vi "File IO - Save Test Parameters to File.vi"(8 "error in":errorcluster, 10 "Experiment Parameter Values (default)":T1(array[cluster]), 11 "start path":path=path "") -> (0 "error out":errorcluster, 3 "selected path":path)   [LabVIEW 2014, in "Core SubVIs.lvlib"]
uses:
  Core SubVIs.lvlib
  Instance           1 46Saved   File IO - Save Test Parameters to File .vi
  <vilib>/Utility/config.llb/Write Key (String).vi
  <vilib>/Utility/config.llb/NI_LVConfig.lvlib
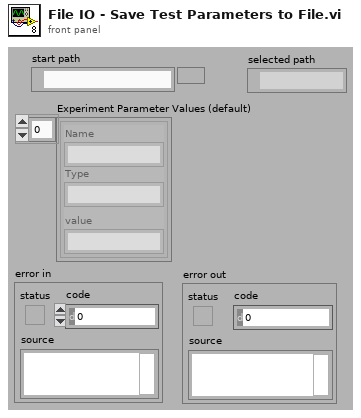
[diagram p1: front panel]
types:
  T1 = cluster{"Name":string, "Type":string, "value":string}[]
  T2 = typedef "NI_LVConfig.lvlib/Config Data RefNum.ctl" = refnum<k1>
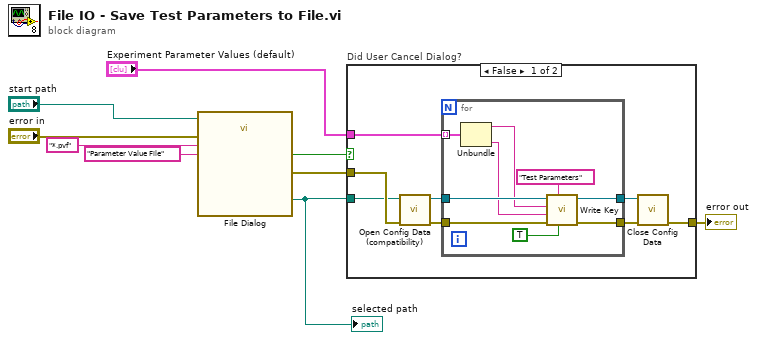
[diagram p0: block diagram]
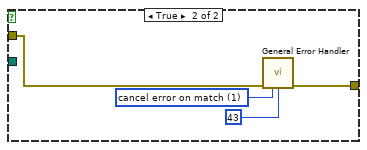
[diagram p2: hidden frame]
diagram:
  n1 = call "File Dialog"("start path"="start path", "error in"="error in", "pattern (all files)"="*.pvf", "pattern label"="Parameter Value File") -> ("selected path"=w6:path, "cancelled"=w5:bool, "error out"=w3:errorcluster)  [unwired: 3 in, 6 out]
  "selected path" <- w6
  n2 = case "Did User Cancel Dialog?" shown="False" w5 {
    tunnel: w6 -> [w15 _]
    tunnel: "Experiment Parameter Values (default)" -> [w17 _]
    tunnel: w3 -> [w16 w30]
    tunnel: [w10 w29] -> w2
    frame False {
      n3 = call <vilib>:"Open Config Data (compatibility).vi"("error in (no error)"=w16, "configuration file path"=w15) -> ("error out"=w13:errorcluster, "refnum"=w14:T2)  [unwired: 7 in, 1 out]
      n4 = for {
        tunnel: w17 -> [w26] mode=indexing
        tunnel: w14 -> [w25]
        tunnel: w13 -> [w24]
        tunnel: [w19] -> w11
        tunnel: [w18] -> w12
        n5 = Unbundle(w26) -> ("Name"=w22:string, "value"=w21:string)  [unwired: 1 out]
        n6 = call-poly <vilib>:"Write Key.vi"("write raw string? (F)"=TRUE, "section"="Test Parameters", "error in (no error)"=w24, "value"=w21, "key"=w22, "refnum"=w25) -> ("error out"=w18:errorcluster, "refnum out"=w19:T2)  [unwired: 4 out]
      }
      n7 = call <vilib>:"Close Config Data.vi"("error in (no error)"=w12, "refnum"=w11) -> ("error out"=w10:errorcluster)  [unwired: 1 in, 8 out]
    }
    frame True {
      w27 = 1 items=["no exception", "cancel error on match", "set error on match"] ("[exception action] (none:0)")
      n8 = call <vilib>:"General Error Handler.vi"("error in (no error)"=w30, "[exception action] (none:0)"=w27, "[exception code]"=43) -> ("error out"=w29:errorcluster)  [unwired: 2 in, 10 out]
    }
  }
  "error out" <- w2
